vi "serialforward.vi"() -> ()   [LabVIEW 2017]
uses:
  <vilib>/Instr/_visa.llb/VISA Configure Serial Port (Instr).vi
panel:
  in  "port":u16=8998
  in  "max buffer size":u32=1000
  in  "parity (0:none)":enum16{"None", "Odd", "Even", "Mark", "Space"}(ring)
  in  "data bits (8)":u16=8 min=5 max=8 step=1
  in  "flow control (0:none)":u16(ring) items=["None", "XON/XOFF", "RTS/CTS", "XON/XOFF & RTS/CTS", "DTR/DSR", "XON/XOFF & DTR/DSR"]
  in  "stop bits (10: 1 bit)":u16(ring)=10 items=["1.0"=10, "1.5"=15, "2.0"=20]
  out "serial error":errorcluster
  in  "termination char\n(0xA = '\\n' = LF)":u8=55 format="%.0x"
  in  "Enable Termination\nChar":bool=TRUE
  in  "baud":u32=115200
  in  "timeout ms":u32=10000
  out "buffer":string
  in  "Port":refnum<visa-resource-name>="COM2"
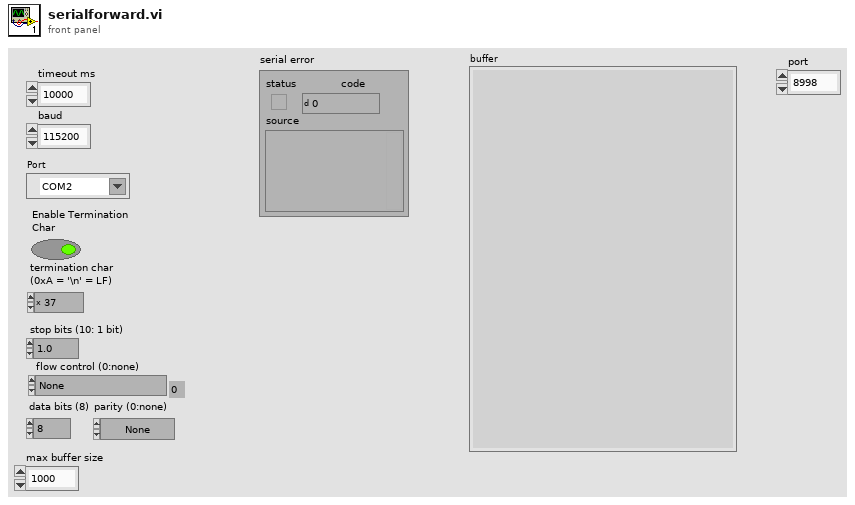
[diagram p1: front panel]
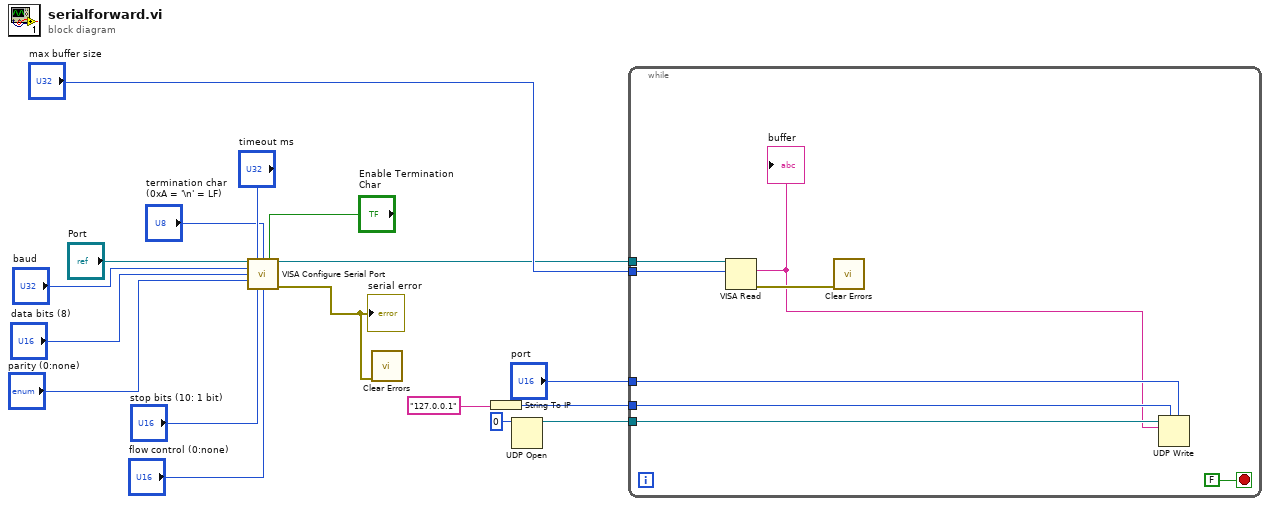
[diagram p0: block diagram]
diagram:
  n1 = call-poly "VISA Configure Serial Port"("VISA resource name"="Port", "timeout (10sec)"="timeout ms", "termination char\n(0xA = '\\n' = LF)"="termination char\n(0xA = '\\n' = LF)", "Enable Termination\nChar (T)"="Enable Termination\nChar", "baud rate (9600)"="baud", "data bits (8)"="data bits (8)", "parity (0:none)"="parity (0:none)", "stop bits (10: 1 bit)"="stop bits (10: 1 bit)", "flow control (0:none)"="flow control (0:none)") -> ("VISA resource name out"=w1:refnum<visa-resource-name>, "error out"=w11:errorcluster)  [unwired: 5 in]
  "serial error" <- w11
  n2 = call <vilib>:"Clear Errors.vi"("error in (no error)"=w11) -> ()  [unwired: 5 in, 2 out]
  n3 = String To IP(1:"127.0.0.1" ("ip")) -> (0:w3:u32)
  n4 = UDP Open(11:u16 0 ("port")) -> (port=w4:refnum<k16>)  [unwired: 4 in, 2 out]
  n5 = while {
    tunnel: "max buffer size" -> [w25]
    tunnel: w4 -> [w24]
    tunnel: w3 -> [w23]
    tunnel: "port" -> [w22]
    tunnel: w1 -> [w20]
    stop <- FALSE stop-if-true
    n6 = VISA Read(VISA resource name=w20, byte count=w25) -> (read buffer=w19:string, error out=w21:errorcluster)  [unwired: 1 in, 2 out]
    "buffer" <- w19
    n7 = call <vilib>:"Clear Errors.vi"("error in (no error)"=w21) -> ()  [unwired: 5 in, 2 out]
    n8 = UDP Write(address=w23, port or service name=w22, connection ID=w24, data in=w19) -> ()  [unwired: 2 in, 2 out]
  }
